vi "dry run for acceleration rate.vi"() -> ()   [LabVIEW 2018]
uses:
  <vilib>/Analysis/1siggen.llb/Ramp Pattern by Delta.vi
  <vilib>/Modbus/master/Modbus Master.lvclass
  <vilib>/Analysis/NI_AALBase.lvlib
  <vilib>/Modbus/master/Create Master Instance (TCP).vi
panel:
  in  "y":bool
  out "Ramp Pattern":dbl[](array[numeric])
  out "Array 2":dbl[][](array[numeric])
  out "Array":dbl[][](array[numeric])
  in  "Stop":dbl
  in  "Start":dbl
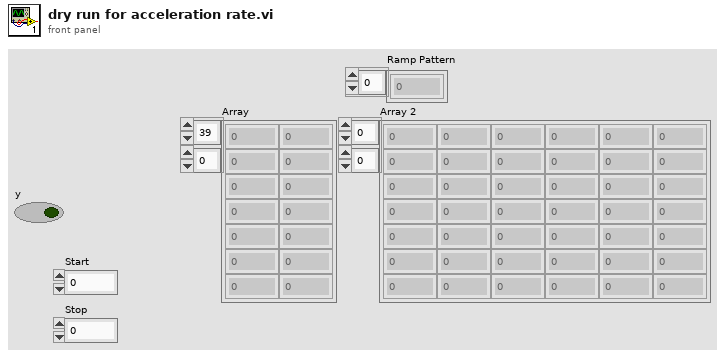
[diagram p1: front panel]
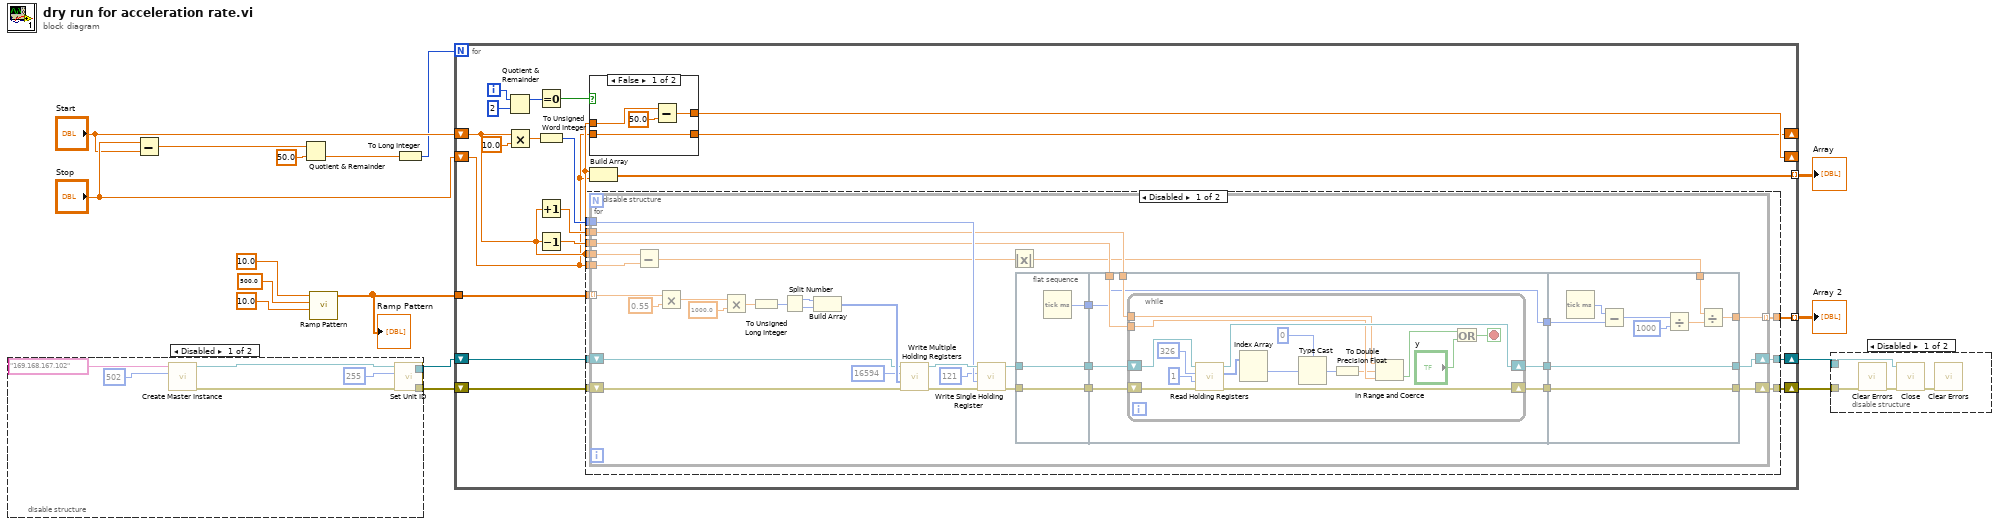
[diagram p0: block diagram]
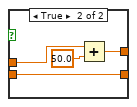
[diagram p5: hidden frame]
diagram:
  n1 = disable-structure shown="Disabled" {
    disable-tunnel: [w18 _] -> w7
    disable-tunnel: [w17 _] -> w6
    frame Disabled {
      n2 = call-poly <vilib>:"Create Master Instance.vi"("port (502)"=u16 502, "address"="169.168.167.102") -> ("error out"=w20:errorcluster, "TCP master instance"=w21:refnum<class "Modbus Master.lvclass">)  [unwired: 8 in]
      n3 = call <vilib>:"Set Unit ID.vi"("error in (no error)"=w20, "unit ID"=u8 255, "Modbus master in"=w21) -> ("error out"=w17:errorcluster, "Modbus master out"=w18:refnum<class "Modbus Master.lvclass">)  [unwired: 7 in]
    }
    frame Enabled {
    }
  }
  n4 = Subtract(x="Stop", y="Start") -> (x-y=w16:dbl)
  n5 = Quotient & Remainder(x=w16, y=50.0) -> (floor(x/y)=w14:dbl)  [unwired: 1 out]
  n6 = call-poly <vilib>:"Ramp Pattern.vi"("start"=10.0, "end"=500.0, "delta"=10.0) -> ("Ramp Pattern"=w5:dbl[])  [unwired: 6 in, 2 out]
  "Ramp Pattern" <- w5
  n7 = To Long Integer(number=w14) -> (32bit integer=w1:i32)
  n8 = for {
    N: w1 -> [_]
    shift-right: [w38] -> _
    shift-left: "Start" -> [w26]
    shift-right: [w39] -> _
    shift-left: "Stop" -> [w25]
    tunnel: [w37] -> w11 mode=indexing
    shift-right: [w33] -> w3
    shift-left: w6 -> [w34]
    tunnel: w5 -> [w36]
    shift-right: [w32] -> w2
    shift-left: w7 -> [w35]
    tunnel: [w24] -> w4 mode=indexing
    i -> [w43]
    n9 = Quotient & Remainder(x=w43, y=2) -> (x-y*floor(x/y)=w41:i32)  [unwired: 1 out]
    n10 = Multiply(x=w26, y=10.0) -> (x*y=w30:dbl)
    n11 = Equal To 0?(x=w41) -> (x = 0?=w40:bool)
    n12 = To Unsigned Word Integer(number=w30) -> (unsigned 16bit integer=w29:u16)
    n13 = Increment(x=w26) -> (x+1=w28:dbl)
    n14 = Decrement(x=w26) -> (x-1=w27:dbl)
    n15 = disable-structure shown="Disabled" {
      disable-tunnel: w36 -> [w54 _]
      disable-tunnel: w35 -> [w53 w124]
      disable-tunnel: w34 -> [w52 w123]
      disable-tunnel: [w51 w123] -> w33
      disable-tunnel: [w50 w124] -> w32
      disable-tunnel: w29 -> [w49 _]
      disable-tunnel: w28 -> [w48 _]
      disable-tunnel: w27 -> [w47 _]
      disable-tunnel: w26 -> [w46 _]
      disable-tunnel: w25 -> [w45 _]
      disable-tunnel: [w44 _] -> w24
      frame Disabled {
        n16 = for {
          tunnel: w54 -> [w80] mode=indexing
          shift-right: [w67] -> w50
          shift-left: w53 -> [w77]
          shift-right: [w66] -> w51
          shift-left: w52 -> [w76]
          tunnel: w49 -> [w71]
          tunnel: w48 -> [w69]
          tunnel: w47 -> [w68]
          tunnel: w46 -> [w59]
          tunnel: w45 -> [w58]
          tunnel: [w55] -> w44 mode=indexing
          n17 = Subtract(x=w59, y=w58) -> (x-y=w57:dbl)
          n18 = Multiply(x=w80, y=0.55) -> (x*y=w78:dbl)
          n19 = Multiply(x=w78, y=1000.0) -> (x*y=w87:dbl)
          n20 = To Unsigned Long Integer(number=w87) -> (unsigned 32bit integer=w86:u32)
          n21 = Split Number(x=w86) -> (hi(x)=w85:u16, lo(x)=w84:u16)
          n22 = Build Array(w85, w84) -> (w83:u16[])
          n23 = call-dynamic "Write Multiple Holding Registers.vi"("error in (no error)"=w76, "holding register values"=w83, "starting address"=u16 16594, "Modbus master in"=w77) -> ("error out"=w74:errorcluster, "Modbus master out"=w75:refnum<class "Modbus Master.lvclass">)  [unwired: 6 in]
          n24 = call-dynamic "Write Single Holding Register.vi"("error in (no error)"=w74, "holding register value"=w71, "address"=u16 121 ("starting address"), "Modbus master in"=w75) -> ("error out"=w72:errorcluster, "Modbus master out"=w73:refnum<class "Modbus Master.lvclass">)  [unwired: 6 in]
          n25 = Absolute Value(x=w57) -> (abs(x)=w56:dbl)
          n26 = flat-sequence {
            tunnel: w72 -> [w89]
            tunnel: w73 -> [w90]
            tunnel: [w90] -> w65
            tunnel: [w89] -> w64
            tunnel: [w88] -> w61
            tunnel: w69 -> [w95]
            tunnel: w68 -> [w94]
            tunnel: w65 -> [w97]
            tunnel: w64 -> [w96]
            tunnel: [w93] -> w63
            tunnel: [w92] -> w62
            tunnel: w61 -> [w91]
            tunnel: [w91] -> w60
            tunnel: [w121] -> w66
            tunnel: [w122] -> w67
            tunnel: w63 -> [w122]
            tunnel: w62 -> [w121]
            tunnel: w60 -> [w119]
            tunnel: w56 -> [w115]
            tunnel: [w114] -> w55
            frame #0 {
              n27 = Tick Count (ms)() -> (millisecond timer value=w88:u32)
            }
            frame #1 {
              n28 = while {
                shift-right: [w106] -> w92
                shift-left: w96 -> [w112]
                shift-right: [w105] -> w93
                shift-left: w97 -> [w113]
                tunnel: w95 -> [w104]
                tunnel: w94 -> [w103]
                stop <- w99 stop-if-true
                n29 = call-dynamic "Read Holding Registers.vi"("error in (no error)"=w112, "number of holding registers"=u16 1, "starting address"=u16 326, "Modbus master in"=w113) -> ("error out"=w106:errorcluster, "register values"=w107:u16[], "Modbus master out"=w105:refnum<class "Modbus Master.lvclass">)  [unwired: 5 in]
                n30 = Index Array(array=w107) -> (element #1=w110:u16)  [unwired: 2 in, 1 out]
                n31 = Type Cast(type=i16 0, x=w110) -> (*(type *) &x=w108:i16)
                n32 = To Double Precision Float(number=w108) -> (double precision float=w102:dbl)
                n33 = In Range and Coerce(upper limit=w104, x=w102, lower limit=w103) -> (In Range?=w101:bool)  [unwired: 1 out]
                n34 = Or(x=w101, y="y") -> (x .or. y?=w99:bool)
              }
            }
            frame #2 {
              n35 = Tick Count (ms)() -> (millisecond timer value=w120:u32)
              n36 = Subtract(x=w120, y=w119) -> (x-y=w118:u32)
              n37 = Divide(x=w118, y=u32 1000) -> (x/y=w116:dbl)
              n38 = Divide(x=w115, y=w116) -> (x/y=w114:dbl)
            }
          }
        }
      }
      frame Enabled {
      }
    }
    n39 = case shown="False" w40 {
      tunnel: w26 -> [w127 w131]
      tunnel: [w125 w130] -> w39
      tunnel: [w128 w129] -> w38
      tunnel: w25 -> [w128 w129]
      frame False {
        n40 = Subtract(x=w127, y=50.0) -> (x-y=w125:dbl)
      }
      frame True {
        n41 = Add(x=w131, y=50.0) -> (x+y=w130:dbl)
      }
    }
    n42 = Build Array(w26, w25) -> (w37:dbl[])
  }
  "Array" <- w11
  "Array 2" <- w4
  n43 = disable-structure shown="Disabled" {
    disable-tunnel: w3 -> [w134 _]
    disable-tunnel: w2 -> [w133 _]
    frame Disabled {
      n44 = call <vilib>:"Clear Errors.vi"("error in (no error)"=w134) -> ("error out"=w135:errorcluster)  [unwired: 5 in, 1 out]
      n45 = call-dynamic "Close.vi"("error in (no error)"=w135, "Modbus master in"=w133) -> ("error out"=w136:errorcluster)  [unwired: 9 in]
      n46 = call <vilib>:"Clear Errors.vi"("error in (no error)"=w136) -> ()  [unwired: 5 in, 2 out]
    }
    frame Enabled {
    }
  }
